vi "APartner.vi"() -> ()   [LabVIEW 2020]
uses:
  lib/Snap7.lvlib
panel:
  out "Data Sent":string
  in  "R__ID":u32=1 format="%08x"
  out "Partner Status":i32(ring) items=["Stopped", "Connecting", "Waiting", "Linked", "Sending", "Receiving", "Bind Error"]
  in  "stop":bool
  in  "TSAP":u16=4098 format="%x"
  in  "Address IP":string="192.168.1.200"
  out "Start Result":string
  in  "TSAP":u16=4098 format="%x"
  in  "Address IP":string="0.0.0.0"
  # "Local"
  # "Remote"
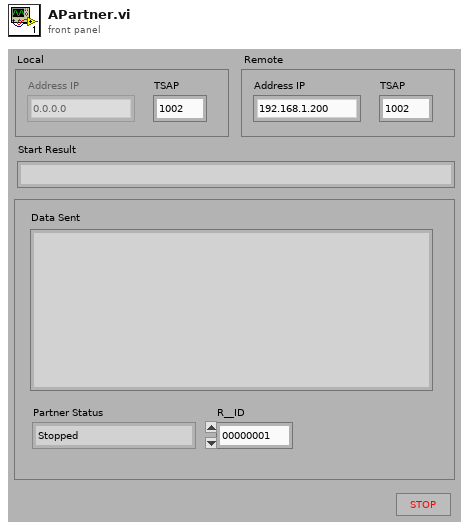
[diagram p1: front panel]
types:
  T1 = enum16{"big-endian, network order", "native, host order", "little-endian"}
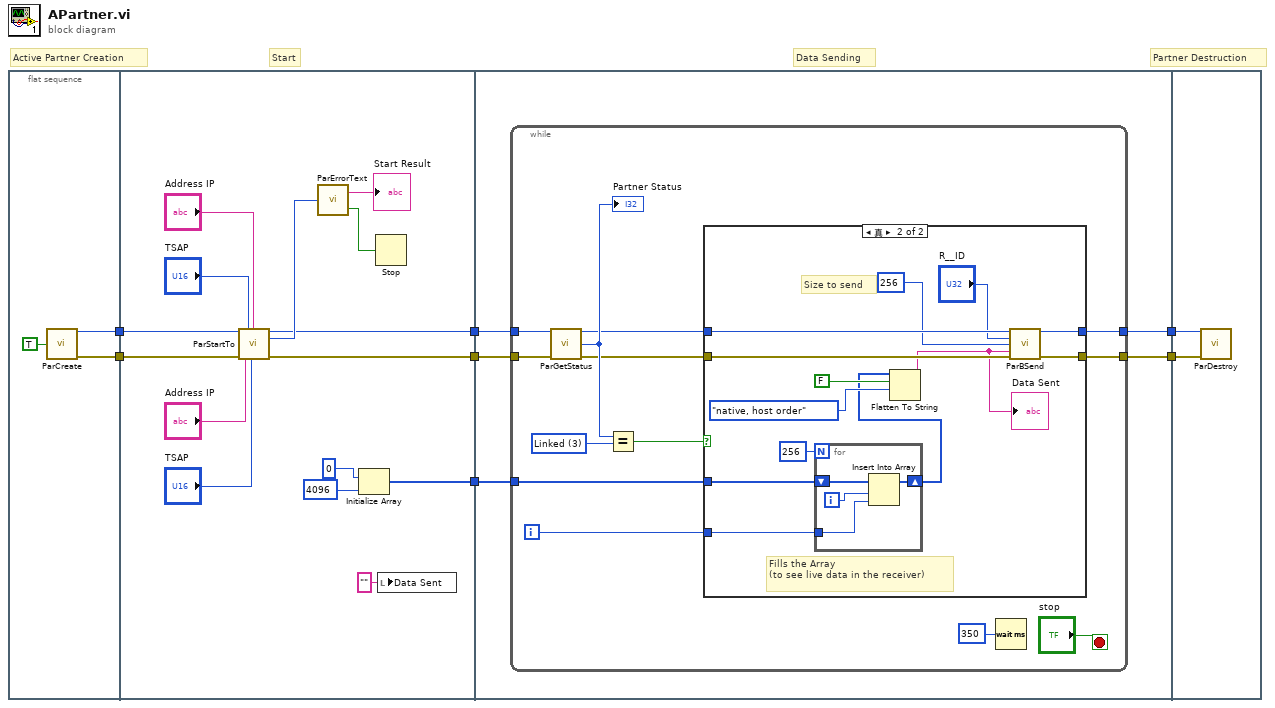
[diagram p0: block diagram]
diagram:
  # "Partner Destruction"
  # "Data Sending"
  # "Start"
  # "Active Partner Creation"
  n1 = flat-sequence {
    tunnel: [w9] -> w7
    tunnel: [w8] -> w6
    tunnel: w7 -> [w23]
    tunnel: w6 -> [w25]
    tunnel: [w16] -> w5
    tunnel: [w15] -> w4
    tunnel: [w12] -> w1
    tunnel: w5 -> [w30]
    tunnel: w4 -> [w29]
    tunnel: [w28] -> w3
    tunnel: [w27] -> w2
    tunnel: w1 -> [w26]
    tunnel: w3 -> [w64]
    tunnel: w2 -> [w63]
    frame #0 {
      n2 = call "ParCreate.vi"("Boolean"=TRUE) -> ("ref out"=w9:u64, "error out"=w8:errorcluster)  [unwired: 13 in]
    }
    frame #1 {
      n3 = call "ParStartTo.vi"("ref in"=w23, "LocalTSAP"="TSAP", "Local Address"="Address IP", "error in (no error)"=w25, "Remote Address"="Address IP", "RemoteTSAP"="TSAP") -> ("ref out"=w16:u64, "Result"=w17:i32, "error out"=w15:errorcluster)  [unwired: 7 in]
      n4 = call "ParErrorText.vi"("ErrNo"=w17) -> ("Error"=w18:bool, "ErrMessage"=→"Start Result":string)
      n5 = Initialize Array(u8 0, 4096) -> (w12:u8[])
      n6 = Stop(stop? (T)=w18) -> ()
      n7 = local write "Data Sent"("" ("Data Sent")) -> ()
    }
    frame #2 {
      n8 = while {
        tunnel: w30 -> [w42]
        tunnel: w29 -> [w41]
        tunnel: [w35] -> w28
        tunnel: [w33] -> w27
        tunnel: w26 -> [w32]
        i -> [w31]
        stop <- "stop" stop-if-true
        w39 = 3 items=["Stopped", "Connecting", "Waiting", "Linked", "Sending", "Receiving", "Bind Error"] ("Partner Status 2")
        n9 = call "ParGetStatus.vi"("ref in"=w42, "error in (no error)"=w41) -> ("ref out"=w36:u64, "Status"=w38:i32, "error out"=w34:errorcluster)  [unwired: 10 in, 1 out]
        "Partner Status" <- w38
        n10 = Equal?(x=w38, y=w39) -> (x = y?=w37:bool)
        n11 = case shown="真" w37 {
          tunnel: w36 -> [w45 w55]
          tunnel: [w45 w53] -> w35
          tunnel: w34 -> [w44 w54]
          tunnel: [w44 w52] -> w33
          tunnel: w32 -> [_ w58]
          tunnel: w31 -> [_ w49]
          frame False {
          }
          frame True {
            # "Size to send"
            # "Fills the Array \n(to see live data in the receiver)"
            n12 = for {
              N: 256 -> [_]
              shift-right: [w60] -> w48
              shift-left: w58 -> [w62]
              tunnel: w49 -> [w59]
              i -> [w61]
              n13 = Insert Into Array(array=w62, index=w61, new element=w59) -> (w60:u8[])
            }
            n14 = Flatten To String(anything=w48, prepend array or string size? (T)=FALSE, byte order (0:big-endian, network order)=T1."native, host order") -> (data string=w46:string)  [unwired: 1 in, 2 out]
            "Data Sent" <- w46
            n15 = call "ParBSend.vi"("ref in"=w55, "R__ID"="R__ID", "Size"=256, "Data"=w46, "error in (no error)"=w54) -> ("ref out"=w53:u64, "error out"=w52:errorcluster)  [unwired: 8 in, 1 out]
          }
        }
        n16 = Wait (ms)(milliseconds to wait=u32 350 ("Loop Delay (ms)")) -> ()  [unwired: 1 out]
      }
    }
    frame #3 {
      n17 = call "ParDestroy.vi"("ref in"=w64, "error in (no error)"=w63) -> ()  [unwired: 13 in, 1 out]
    }
  }
